vi "Handle Measure RPC.vi"(7 "reentrant":bool=TRUE, 9 "measurement plugin service in":refnum<class "Measurement Plugin Service.lvclass">, 10 "gRPC ID in":T1, 11 "measurement service in":refnum<class "IMeasurement Service.lvclass">) -> ()   [LabVIEW 2021, in "NI Measurement Plug-In SDK.lvlib" / "IMeasurement Service.lvclass"]
uses:
  IMeasurement Service.lvclass
  <vilib>/gRPC/LabVIEW gRPC Library/Shared/grpcId.ctl
  Measurement Plugin Service/Measurement Plugin Service.lvclass
  gRPC/Generated APIs/ni/measurementlink/measurement/v2/RPC Service/MeasurementService/MeasurementServiceBaseV2.lvclass
  <vilib>/gRPC/LabVIEW gRPC Library/grpc-lvsupport-release.lvlib
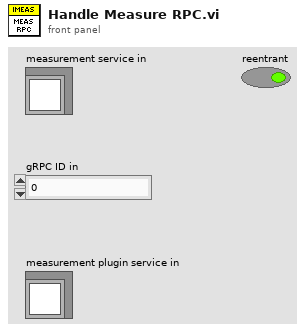
[diagram p1: front panel]
types:
  T1 = typedef "grpc-lvsupport-release.lvlib/grpcId.ctl" = u64
  T2 = typedef "ni.measurementlink.measurement.v2.api.lvlib/ni_measurementlink_measurement_v2_MeasureRequest.ctl" = cluster{"configuration_parameters":T3, "pin_map_context":T4}
  T3 = typedef "ni.measurementlink.measurement.v2.api.lvlib/google_protobuf_Any.ctl" = cluster{"type_url":string, "value":u8[]}
  T4 = typedef "ni.measurementlink.measurement.v2.api.lvlib/ni_measurementlink_PinMapContext.ctl" = cluster{"pin_map_id":string, "sites":i32[]}
  T5 = typedef "NI Measurement Plug-In SDK.lvlib/Measure Response.ctl" = cluster{"outputs":T6}
  T6 = typedef "ni.measurementlink.measurement.v1.api.lvlib/google_protobuf_Any.ctl" = cluster{"type_url":string, "value":u8[]}
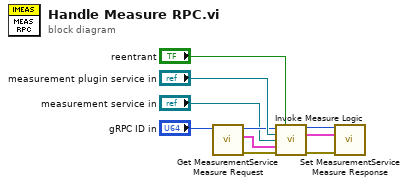
[diagram p0: block diagram]
diagram:
  n1 = call "Get MeasurementService Measure Request.vi"("gRPCid"="gRPC ID in") -> ("error out"=w8:errorcluster, "Message Data"=w9:T2, "gRPCid out"=w4:T1)  [unwired: 8 in]
  n2 = call "Invoke Measure Logic.vi"("gRPC ID in"=w4, "reentrant"="reentrant", "measurement plugin service in"="measurement plugin service in", "measurement service in"="measurement service in", "measure request"=w9, "error in"=w8) -> ("gRPC ID out"=w3:T1, "measure response"=w7:T5, "error out"=w5:errorcluster)  [unwired: 7 in]
  n3 = call "Set MeasurementService Measure Response.vi"("error in (no error)"=w5, "Message Data"=w7, "gRPCid in"=w3) -> ()  [unwired: 8 in, 1 out]
